vi "VariantAttributeExample.vi"() -> ()   [LabVIEW 2025]
doc: "Author: Scott Hannahs <sth@magnet.fsu.edu>\n\nThis software is licensed for use under the “MIT License\"\nCopyright (c) 2025 Scott Hannahs, sth@sth@magnet.sthnet.net\n\nPermission is hereby granted, free of charge, to any person obtaining a copy of this software and associated documentation files (the \"Software\"), to deal in the Software without restriction, including without limitation the rights to use, copy, modify, merge, publish, distribute, sublicense, and/or sell copies of the Software, and to permit persons to whom the Software is furnished to do so, subject to the following conditions: The above copyright notice and this permission notice shall be included in all copies or substantial portions of the Software.\n\nTHE SOFTWARE IS PROVIDED \"AS IS\", WITHOUT WARRANTY OF ANY KIND, EXPRESS OR IMPLIED, INCLUDING BUT NOT LIMITED TO THE WARRANTIES OF MERCHANTABILITY, FITNESS FOR A PARTICULAR PURPOSE AND NONINFRINGEMENT. IN NO EVENT SHALL THE AUTHORS OR COPYRIGHT HOLDERS BE LIABLE FOR ANY CLAIM, DAMAGES OR OTHER LIABILITY, WHETHER IN AN ACTION OF CONTRACT, TORT OR OTHERWISE, ARISING FROM, OUT OF OR IN CONNECTION WITH THE SOFTWARE OR THE USE OR OTHER DEALINGS IN THE SOFTWARE."
panel:
  out "names":string[](array[string])
  out "values 2":variant[](array[variant])
  in  "Array":cluster{bool, i32}[](array[cluster])=[{FALSE, 0}, {TRUE, 123}, {FALSE, 234}]
  out "values":cluster{bool, i32}
  in  "Object to Get":T1(ring)
  # "Simply select an object to get and press run. Note\nhow the output corresponds to the cluster values\nwe are \"storing\" by name in the variant as Variant\nAttributes"
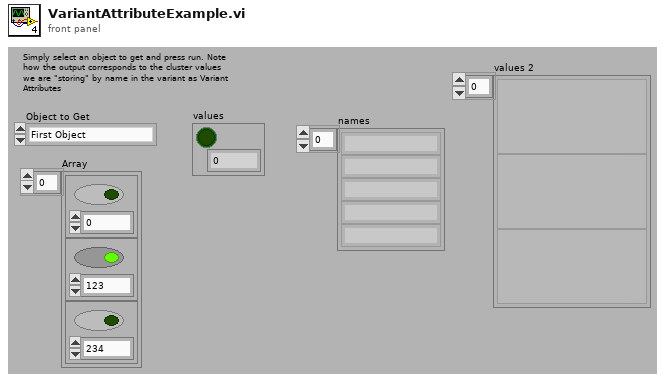
[diagram p1: front panel]
types:
  T1 = enum16{"First Object", "Second Object", "Third Object"}
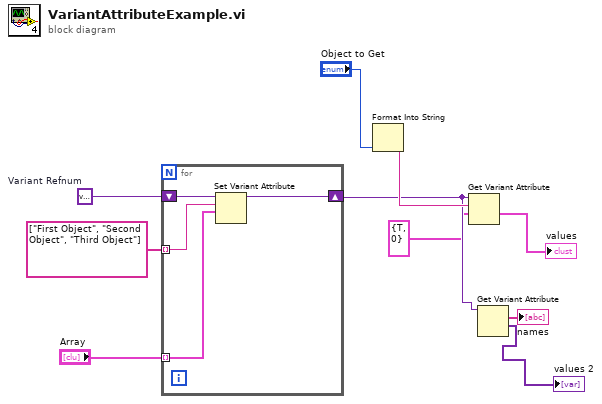
[diagram p0: block diagram]
diagram:
  w10 = variant  # Variant Refnum
  n1 = for {
    shift-right: [w13] -> w4
    shift-left: w10 -> [w14]
    tunnel: string[] ["First Object", "Second Object", "Third Object"] -> [w12] mode=indexing
    tunnel: "Array" -> [w11] mode=indexing
    n2 = Set Variant Attribute(Variant=w14, name=w12, value=w11) -> (Variant out=w13:variant)  [unwired: 1 in, 2 out]
  }
  n3 = Format Into String("Object to Get") -> (resulting string=w6:string)  [unwired: 3 in, 1 out]
  n4 = Get Variant Attribute(Variant=w4, name=w6, default value (empty Variant)=cluster{bool, i32} {TRUE, 0}) -> (value=→"values":cluster{bool, i32})  [unwired: 1 in, 3 out]
  n5 = Get Variant Attribute(Variant=w4) -> (names=→"names":string[], values=→"values 2":variant[])  [unwired: 3 in, 2 out]
